vi "Prax13y3.vi"() -> ()   [LabVIEW 2020]
panel:
  out "Data 2":dbl(graph)
  out "Data 1":i32(graph)
  in  "Stop":bool
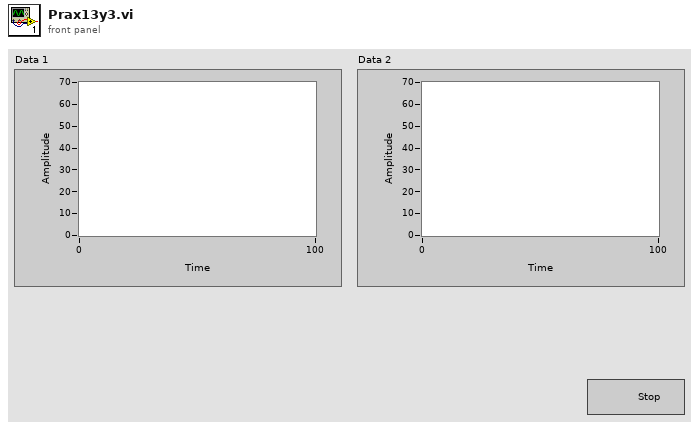
[diagram p1: front panel]
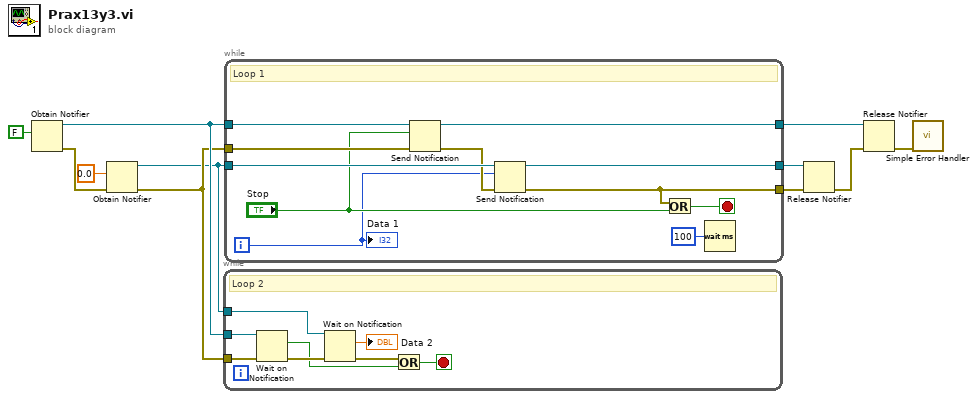
[diagram p0: block diagram]
diagram:
  n1 = Obtain Notifier(notification data type=FALSE) -> (notifier out=w11:refnum<notifier>, error out=w9:errorcluster)  [unwired: 3 in, 1 out]
  n2 = Obtain Notifier(notification data type=0.0, error in (no error)=w9) -> (notifier out=w1:refnum<notifier>, error out=w2:errorcluster)  [unwired: 2 in, 1 out]
  n3 = while {
    tunnel: w11 -> [w18]
    tunnel: w2 -> [w19]
    tunnel: w1 -> [w16]
    stop <- w12 stop-if-true
    # "Loop 2"
    n4 = Wait on Notification(notifier=w18, error in (no error)=w19) -> (notification=w13:bool, error out=w17:errorcluster)  [unwired: 2 in, 2 out]
    n5 = Wait on Notification(notifier=w16, error in (no error)=w17) -> (notification=→"Data 2":dbl, error out=w14:errorcluster)  [unwired: 2 in, 2 out]
    n6 = Or(x=w14, y=w13) -> (x .or. y?=w12:bool)
  }
  n7 = while {
    tunnel: w11 -> [w29]
    tunnel: w2 -> [w28]
    tunnel: [w27] -> w4
    tunnel: w1 -> [w26]
    tunnel: [w24] -> w6
    tunnel: [w23] -> w7
    i -> [w20]
    stop <- w21 stop-if-true
    # "Loop 1"
    n8 = Send Notification(notification="Stop", notifier=w29, error in (no error)=w28) -> (notifier out=w27:refnum<notifier>, error out=w25:errorcluster)
    n9 = Send Notification(notification=w20, notifier=w26, error in (no error)=w25) -> (notifier out=w24:refnum<notifier>, error out=w23:errorcluster)
    n10 = Or(x=w23, y="Stop") -> (x .or. y?=w21:bool)
    n11 = Wait (ms)(milliseconds to wait=u32 100) -> ()  [unwired: 1 out]
    "Data 1" <- w20
  }
  n12 = Release Notifier(notifier=w6, error in (no error)=w7) -> (error out=w5:errorcluster)  [unwired: 1 in, 2 out]
  n13 = Release Notifier(notifier=w4, error in (no error)=w5) -> (error out=w3:errorcluster)  [unwired: 1 in, 2 out]
  n14 = call <vilib>:"Simple Error Handler.vi"("error in (no error)"=w3) -> ()  [unwired: 4 in, 5 out]
